vi "Golander pump example.vi"() -> ()   [LabVIEW 2015]
uses:
  modbusrtu/MB Serial Master Query Write Single Register (poly).vi
panel:
  in  "Serial Parameters":T1={"Mode"=enum."RTU", "Slave Address"=1} {"Slave Address" format="%.0x"}
  in  "speed":u16
  in  "VISA resource name":refnum<visa-resource-name>
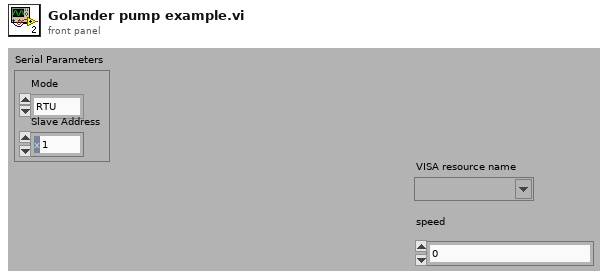
[diagram p1: front panel]
types:
  T1 = cluster{"Mode":enum16{"RTU", "ASCII"}, "Slave Address":u8}
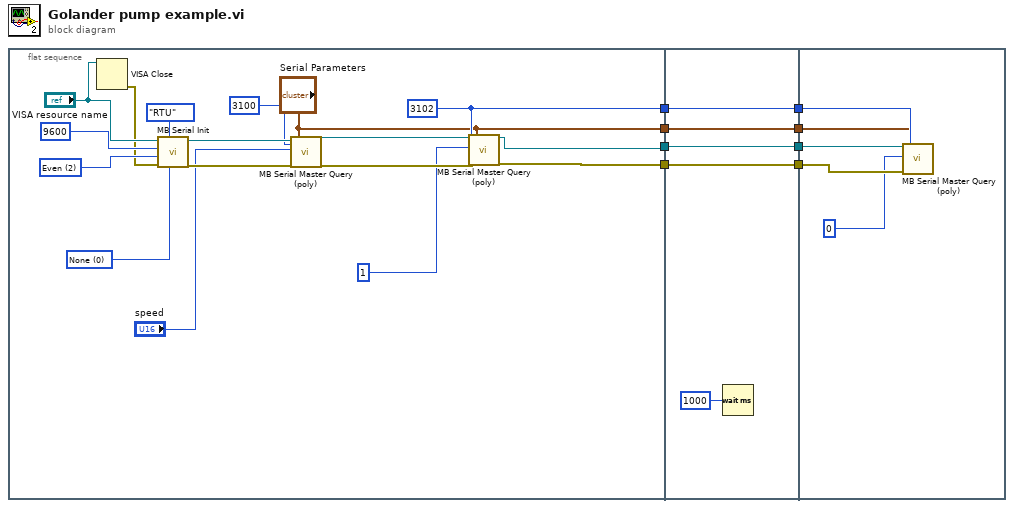
[diagram p0: block diagram]
diagram:
  n1 = flat-sequence {
    tunnel: [w16] -> w7
    tunnel: [w15] -> w6
    tunnel: [w14] -> w4
    tunnel: ["Serial Parameters"] -> w1
    tunnel: [w29] -> w8
    tunnel: w7 -> [w29]
    tunnel: w6 -> [w28]
    tunnel: [w28] -> w5
    tunnel: w4 -> [w27]
    tunnel: [w27] -> w3
    tunnel: [w26] -> w2
    tunnel: w1 -> [w26]
    tunnel: w8 -> [w35]
    tunnel: w5 -> [w34]
    tunnel: w3 -> [w33]
    tunnel: w2 -> [w31]
    frame #0 {
      w14 = u16 3102 ("Address")
      w22 = u16 0 items=["None", "XON/XOFF", "RTS/CTS", "XON/XOFF & RTS/CTS", "DTR/DSR", "XON/XOFF & DTR/DSR"] ("Flow Control")
      w24 = u16 2 items=["None", "Odd", "Even", "Mark", "Space"] ("Parity")
      n2 = VISA Close(VISA resource name="VISA resource name") -> (error out=w9:errorcluster)  [unwired: 1 in]
      n3 = call "MB Serial Init.vi"("Flow Control"=w22, "Mode"=enum16{"RTU", "ASCII"}."RTU", "error in (no error)"=w9, "Parity"=w24, "Baud Rate"=u32 9600, "VISA resource name"="VISA resource name") -> ("error out"=w20:errorcluster, "VISA resource name out"=w21:refnum<visa-resource-name>)  [unwired: 4 in]
      n4 = call-poly "MB Serial Master Query (poly).vi"("VISA resource name"=w21, "Address"=u16 3100, "Holding Register"="speed", "error in"=w20, "Serial Parameters"="Serial Parameters") -> ("VISA resource name out"=w12:refnum<visa-resource-name>, "error out"=w18:errorcluster)  [unwired: 12 in, 1 out]
      n5 = call-poly "MB Serial Master Query (poly).vi"("VISA resource name"=w12, "Address"=w14, "Holding Register"=u16 1, "error in"=w18, "Serial Parameters"="Serial Parameters") -> ("VISA resource name out"=w16:refnum<visa-resource-name>, "error out"=w15:errorcluster)  [unwired: 12 in, 1 out]
    }
    frame #1 {
      n6 = Wait (ms)(milliseconds to wait=u32 1000 ("等待时间（毫秒）")) -> ()  [unwired: 1 out]
    }
    frame #2 {
      n7 = call-poly "MB Serial Master Query (poly).vi"("VISA resource name"=w35, "Address"=w33, "Holding Register"=u16 0, "error in"=w34, "Serial Parameters"=w31) -> ()  [unwired: 12 in, 3 out]
    }
  }
